vi "Dynamixel XL320 Send Advanced Commands.vi"() -> ()   [LabVIEW 2015]
doc: "This example allows you to use all of the available command types for the Dynamixel motor. Refer to the motor's documentation for more information."
uses:
  <instrlib>/Dynamixel XL320/Public/Motor Operation/Low Level/XL320_Baud Setting.ctl
  <instrlib>/Dynamixel XL320/Public/Configure/XL320_Select_Action.ctl
  <instrlib>/Dynamixel XL320/Dynamixel XL320.lvlib
panel:
  in  "Select Action":T1=1 items=["Ping"=1, "Read"=2, "Write"=3, "Registered Write"=4, "Action"=5, "Reset"=6, "Reboot"=8, "Status"=85, "Sync Read"=130, "Sync Write"=131, "Bulk Read"=146, "Bulk Write"=147]
  in  "Baud rate (1,000,000 bps)":T2=3 items=["9600 bps", "57600 bps", "115200 bps", "1,000,000 bps"]
  in  "Force Baud Rate (True)":bool
  out "Last command sent":string
  in  "VISA resource name":refnum<visa-resource-name>
  in  "stop":bool
  out "Responses":string
  in  "Send Command":bool
  in  "Parameters (Hex)":string
  in  "Address":u8
  in  "Motor ID":u8
  in  "Clear":bool
  # "Ghislain REMY, IUT de Cachan, 2015 December 2015"
  # "This example allows you to use all of the available command types for the \nDynamixel XL320.  Refer to the motor's documentation for more information."
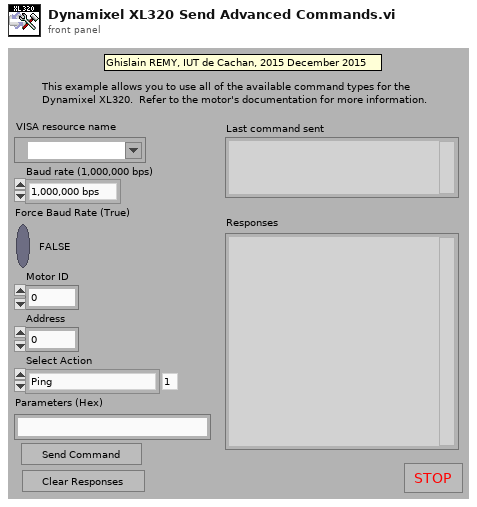
[diagram p1: front panel]
types:
  T1 = typedef "Dynamixel XL320.lvlib/XL320_Select_Action.ctl" = u8
  T2 = typedef "Dynamixel XL320.lvlib/XL320_Baud Setting.ctl" = u8
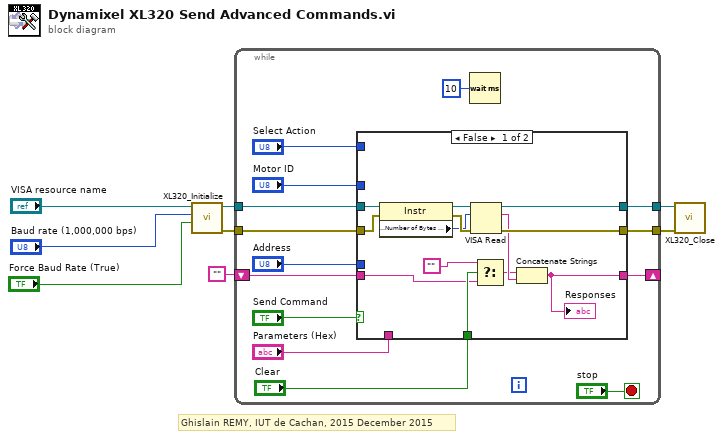
[diagram p0: block diagram]
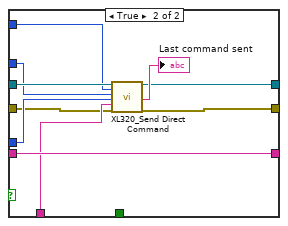
[diagram p2: hidden frame]
diagram:
  # "Ghislain REMY, IUT de Cachan, 2015 December 2015"
  n1 = call <instrlib>:"XL320_Initialize.vi"("Force Baud Rate (True)"="Force Baud Rate (True)", "Baud rate (1,000,000 bps)"="Baud rate (1,000,000 bps)", "VISA resource name"="VISA resource name") -> ("error out"=w5:errorcluster, "VISA resource name out"=w4:refnum<visa-resource-name>)  [unwired: 7 in]
  n2 = while {
    tunnel: w4 -> [w22]
    tunnel: [w21] -> w3
    tunnel: w5 -> [w20]
    tunnel: [w19] -> w2
    shift-right: [w11] -> _
    shift-left: "" -> [w10]
    stop <- "stop" stop-if-true
    n3 = case shown="False" "Send Command" {
      tunnel: w22 -> [w35 w44]
      tunnel: [w30 w36] -> w21
      tunnel: w20 -> [w34 w39]
      tunnel: [w29 w38] -> w19
      tunnel: "Parameters (Hex)" -> [_ w40]
      tunnel: "Address" -> [_ w41]
      tunnel: "Motor ID" -> [_ w42]
      tunnel: "Clear" -> [w27 _]
      tunnel: "Select Action" -> [_ w43]
      tunnel: [w24 w45] -> w11
      tunnel: w10 -> [w23 w45]
      frame False {
        n4 = property class="Instr"(reference=w35, error in=w34) -> (reference out=w31:refnum<visa-resource-name>, error out=w33:errorcluster, "Serial Settings:Number of Bytes at Serial Port"=w32:u32)
        n5 = VISA Read(VISA resource name=w31, byte count=w32, error in (no error)=w33) -> (VISA resource name out=w30:refnum<visa-resource-name>, read buffer=w28:string, error out=w29:errorcluster)  [unwired: 1 out]
        n6 = Select(t="", s=w27, f=w23) -> (s? t:f=w26:string)
        n7 = Concatenate Strings(w26, w28) -> (w24:string)
        "Responses" <- w24
      }
      frame True {
        n8 = call <instrlib>:"XL320_Send Direct Command.vi"("VISA resource name"=w44, "Select Action"=w43, "Motor ID (0)"=w42, "Address"=w41, "Parameters"=w40, "Error in (no error)"=w39) -> ("VISA resource name out"=w36:refnum<visa-resource-name>, "Command to Serial"=→"Last command sent":string, "Error out"=w38:errorcluster)  [unwired: 11 in]
      }
    }
    n9 = Wait (ms)(milliseconds to wait=u32 10) -> ()  [unwired: 1 out]
  }
  n10 = call <instrlib>:"XL320_Close.vi"("error in (no error)"=w2, "VISA resource name"=w3) -> ()  [unwired: 9 in, 1 out]
